vi "TranslateGrpcError.vi"(8 "error in":errorcluster, 10 "Error Message":string, 11 "Error Code":i32) -> (0 "error out":errorcluster)   [LabVIEW 2019, in "grpc-lvsupport.lvlib"]
uses:
  grpc-lvsupport.lvlib
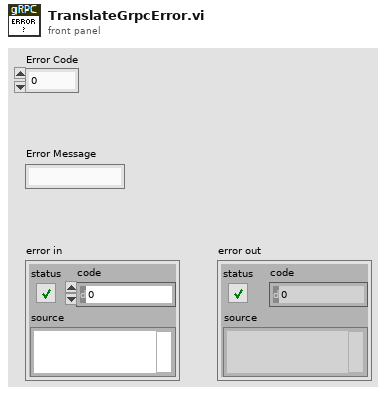
[diagram p1: front panel]
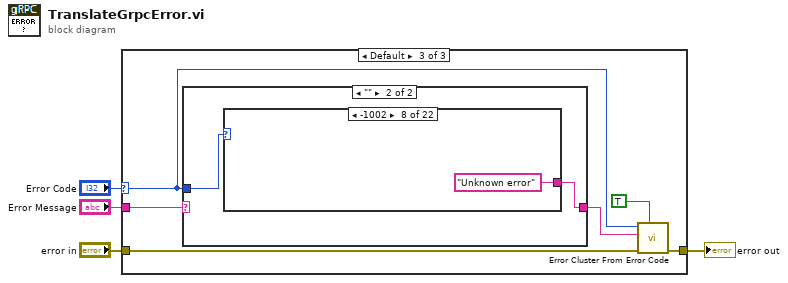
[diagram p0: block diagram]
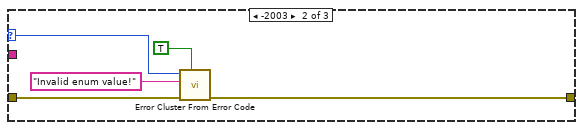
[diagram p3: hidden frame]
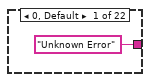
[diagram p5: hidden frame]
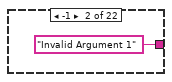
[diagram p6: hidden frame]
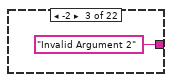
[diagram p7: hidden frame]
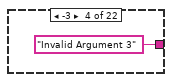
[diagram p8: hidden frame]
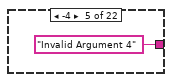
[diagram p9: hidden frame]
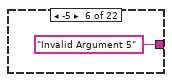
[diagram p10: hidden frame]
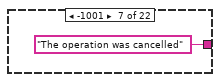
[diagram p11: hidden frame]
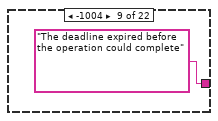
[diagram p12: hidden frame]
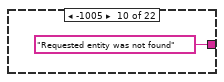
[diagram p13: hidden frame]
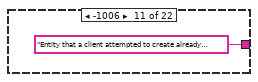
[diagram p14: hidden frame]
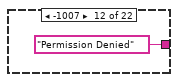
[diagram p15: hidden frame]
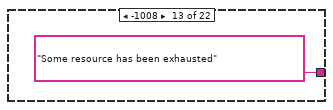
[diagram p16: hidden frame]
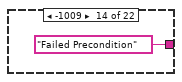
[diagram p17: hidden frame]
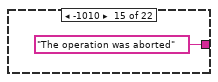
[diagram p18: hidden frame]
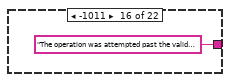
[diagram p19: hidden frame]
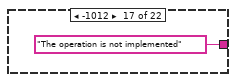
[diagram p20: hidden frame]
diagram:
  n1 = case shown="Default" "Error Code" {
    selector: "Error Code" -> [_ w8 w14]
    tunnel: [w5 w7 w12] -> w2
    tunnel: "Error Message" -> [_ _ w16]
    tunnel: "error in" -> [w5 w6 w11]
    frame 0 {
    }
    frame -2003 {
      n2 = call <vilib>:"Error Cluster From Error Code.vi"("show call chain? (False)"=TRUE, "error in (no error)"=w6, "error message (\"\")"="Invalid enum value!" ("error source (\" \")"), "error code (0)"=w8) -> ("error out"=w7:errorcluster)  [unwired: 5 in]
    }
    frame Default {
      n3 = case shown="\"\"" w16 {
        selector: w16 -> [w17 _]
        tunnel: w14 -> [_ w19]
        tunnel: [w17 w18] -> w15
        frame Default {
        }
        frame "" {
          n4 = case shown="-1002" w19 {
            tunnel: ["Unknown Error" "Invalid Argument 1" "Invalid Argument 2" "Invalid Argument 3" "Invalid Argument 4" "Invalid Argument 5" "The operation was cancelled" "Unknown error" "The deadline expired before the operation could complete" "Requested entity was not found" "Entity that a client attempted to create already exists" "Permission Denied" "Some resource has been exhausted" "Failed Precondition" "The operation was aborted" "The operation was attempted past the valid range" "The operation is not implemented" "Internal error" "The service is currently unavailable" "Unrecoverable data loss or corruption" "The request does not have valid authentication credentials" "The client specified an invalid argument"] -> w18
            frame 0, Default {
            }
            frame -1 {
            }
            frame -2 {
            }
            frame -3 {
            }
            frame -4 {
            }
            frame -5 {
            }
            frame -1001 {
            }
            frame -1002 {
            }
            frame -1004 {
            }
            frame -1005 {
            }
            frame -1006 {
            }
            frame -1007 {
            }
            frame -1008 {
            }
            frame -1009 {
            }
            frame -1010 {
            }
            frame -1011 {
            }
            frame -1012 {
            }
            frame -1013 {
            }
            frame -1014 {
            }
            frame -1015 {
            }
            frame -1016 {
            }
            frame -1003 {
            }
          }
        }
      }
      n5 = call <vilib>:"Error Cluster From Error Code.vi"("show call chain? (False)"=TRUE, "error in (no error)"=w11, "error message (\"\")"=w15, "error code (0)"=w14) -> ("error out"=w12:errorcluster)  [unwired: 5 in]
    }
  }
  "error out" <- w2
